vi "test-globallog for CSM error.vi"(8 "error in (no error)":errorcluster, 11 "TestCase in":refnum<class "testcase-globalLog.lvclass">) -> (0 "error out":errorcluster, 3 "TestCase out":refnum<class "testcase-globalLog.lvclass">)   [LabVIEW 2017, in "testcase-globalLog.lvclass"]
uses:
  testcase-globalLog.lvclass
  src/user.lib/_NEVSTOP/Communicable State Machine(CSM)/_Support/Priority Queue/Priority Queue.lvclass/Priority Queue.ctl
  src/user.lib/_NEVSTOP/Communicable State Machine(CSM)/_Support/Typedef/_CSM_GlobalLog_MSG.ctl
  src/user.lib/_NEVSTOP/Communicable State Machine(CSM)/_Support/Typedef/_CSM_Response Source Message.ctl
  src/user.lib/_NEVSTOP/Communicable State Machine(CSM)/_Support/Typedef/_CSM_GlobalLog_MSG_TYPE.ctl
  61f80922-628e-48dd-9b7e-09b6add618c8.vi
  src/user.lib/_NEVSTOP/Communicable State Machine(CSM)/_Support/GlobalEvent/Gevt-ThreadQueueName.vi
  src/user.lib/_NEVSTOP/Communicable State Machine(CSM)/_Support/Process/CSMP-Sync Call.vi
  src/user.lib/_NEVSTOP/Communicable State Machine(CSM)/Utility/uuid.vi
  src/user.lib/_NEVSTOP/Communicable State Machine(CSM)/Utility/Build Error Cluster.vi
  src/user.lib/_NEVSTOP/Communicable State Machine(CSM)/Utility/Trim Both Whitespace.vi
  src/user.lib/_NEVSTOP/Communicable State Machine(CSM)/_Support/CSMQ/_CSMObj-Message Check.vi
  src/user.lib/_NEVSTOP/Communicable State Machine(CSM)/_Support/CSMQ/_CSMObj-Enqueue Cross-Module Message.vi
  src/user.lib/_NEVSTOP/Communicable State Machine(CSM)/_Support/CSMQ/_CSMOFGV Get.vi
  src/user.lib/_NEVSTOP/Communicable State Machine(CSM)/_Support/Priority Queue/Enqueue Element.vi
  src/user.lib/_NEVSTOP/Communicable State Machine(CSM)/_Support/FGV-BroadcastRegistry/global-CSMQ FGV Change Flag.vi
  src/user.lib/_NEVSTOP/Communicable State Machine(CSM)/_Support/CSMQ/_CSMOFGV.vi
  src/user.lib/_NEVSTOP/Communicable State Machine(CSM)/_Support/Error/CSM No Target Error.vi
  src/user.lib/_NEVSTOP/Communicable State Machine(CSM)/_Support/Error/CSM Not Allowed Message.vi
  src/user.lib/_NEVSTOP/Communicable State Machine(CSM)/_Support/Error/CSM Target Error.vi
  src/user.lib/_NEVSTOP/Communicable State Machine(CSM)/_Support/Error/CSM Unhandled State Error.vi
  src/user.lib/_NEVSTOP/Communicable State Machine(CSM)/_Support/Error/CSM Target Timeout Error.vi
  <vilib>/addons/_JKI Toolkits/VI Tester/TestCase.llb/TestCase.lvclass
  src/user.lib/_NEVSTOP/Communicable State Machine(CSM)/Communicable State Machine.lvlib
  C:/Program Files (x86)/National Instruments/LabVIEW 2017/vi.lib/addons/_JKI Toolkits/VI Tester/TestCase.llb/TestCase.lvclass
panel:
  out "State History":string
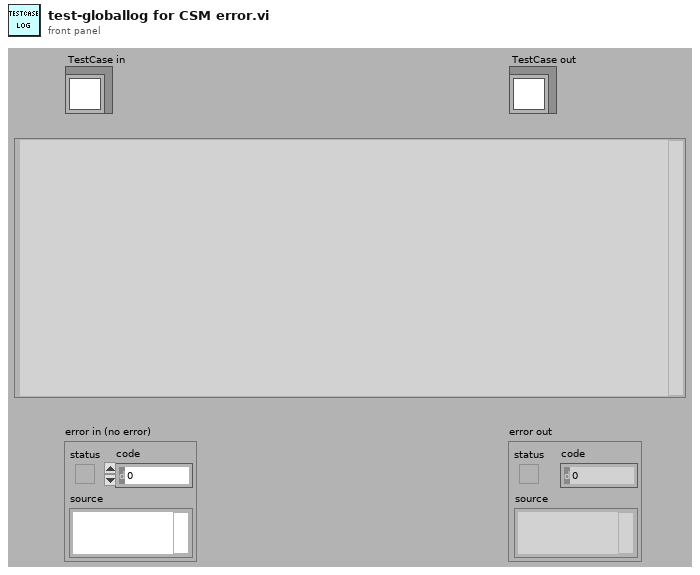
[diagram p1: front panel]
types:
  T1 = cluster{"threashold(#/s)":dbl, "Check Peroid(s)":dbl}
  T2 = typedef "Communicable State Machine.lvlib/_CSM_GlobalLog_MSG.ctl" = cluster{"Name(\"\" to use uuid)":string, "Current State":string, "Arguments":string, "Source Message":T3, "Source Module":string, "Complete(T)/Start(F)":bool, "LogType":T4}
  T3 = typedef "Communicable State Machine.lvlib/_CSM_Response Source Message.ctl" = cluster{"‘State":string, "’Arguments":string, "’Error":errorcluster}
  T4 = typedef "Communicable State Machine.lvlib/_CSM_GlobalLog_MSG_TYPE.ctl" = enum16{"User Log", "State Change", "Status", "Interrupt", "Register", "Unregister", "Error Log", "Module Created", "Module Destroyed"}
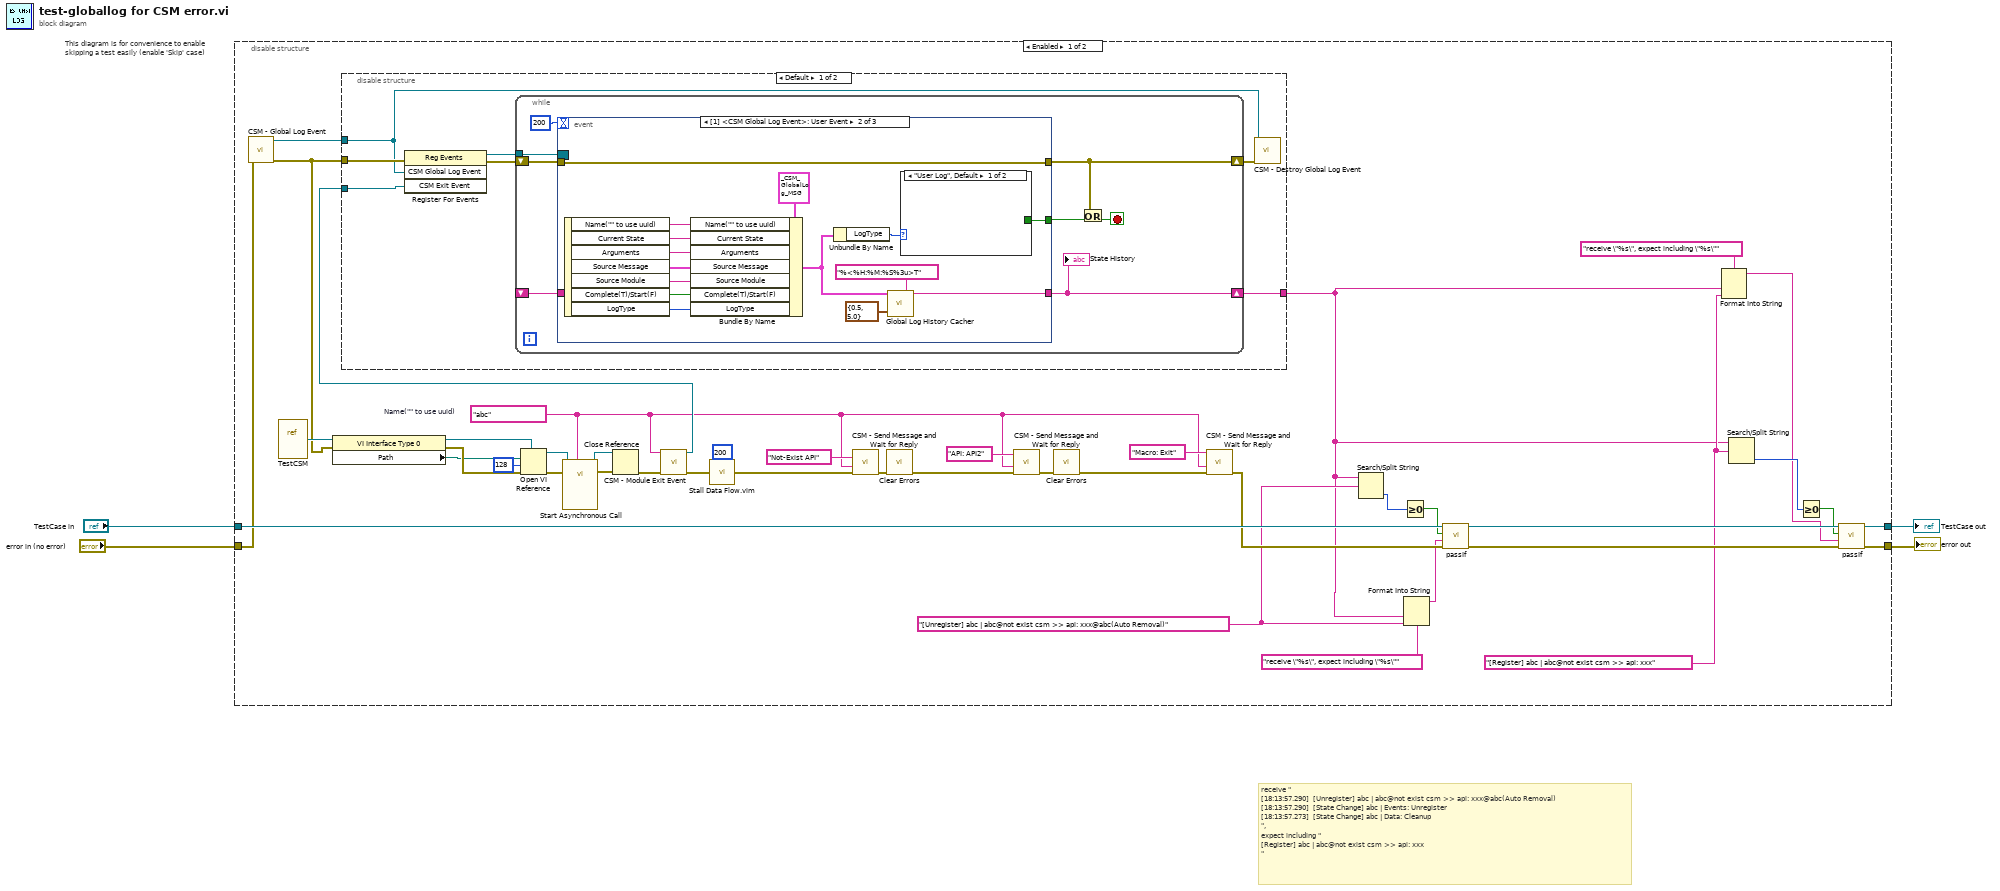
[diagram p0: block diagram]
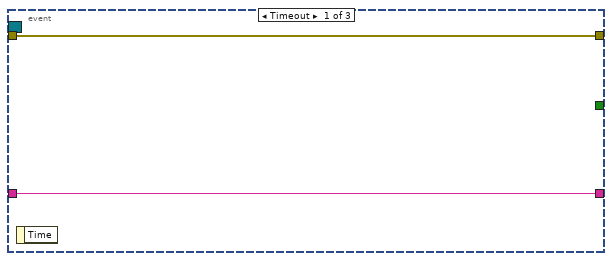
[diagram p2: hidden frame]
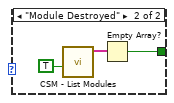
[diagram p3: hidden frame]
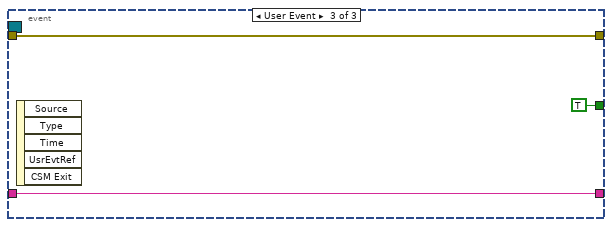
[diagram p4: hidden frame]
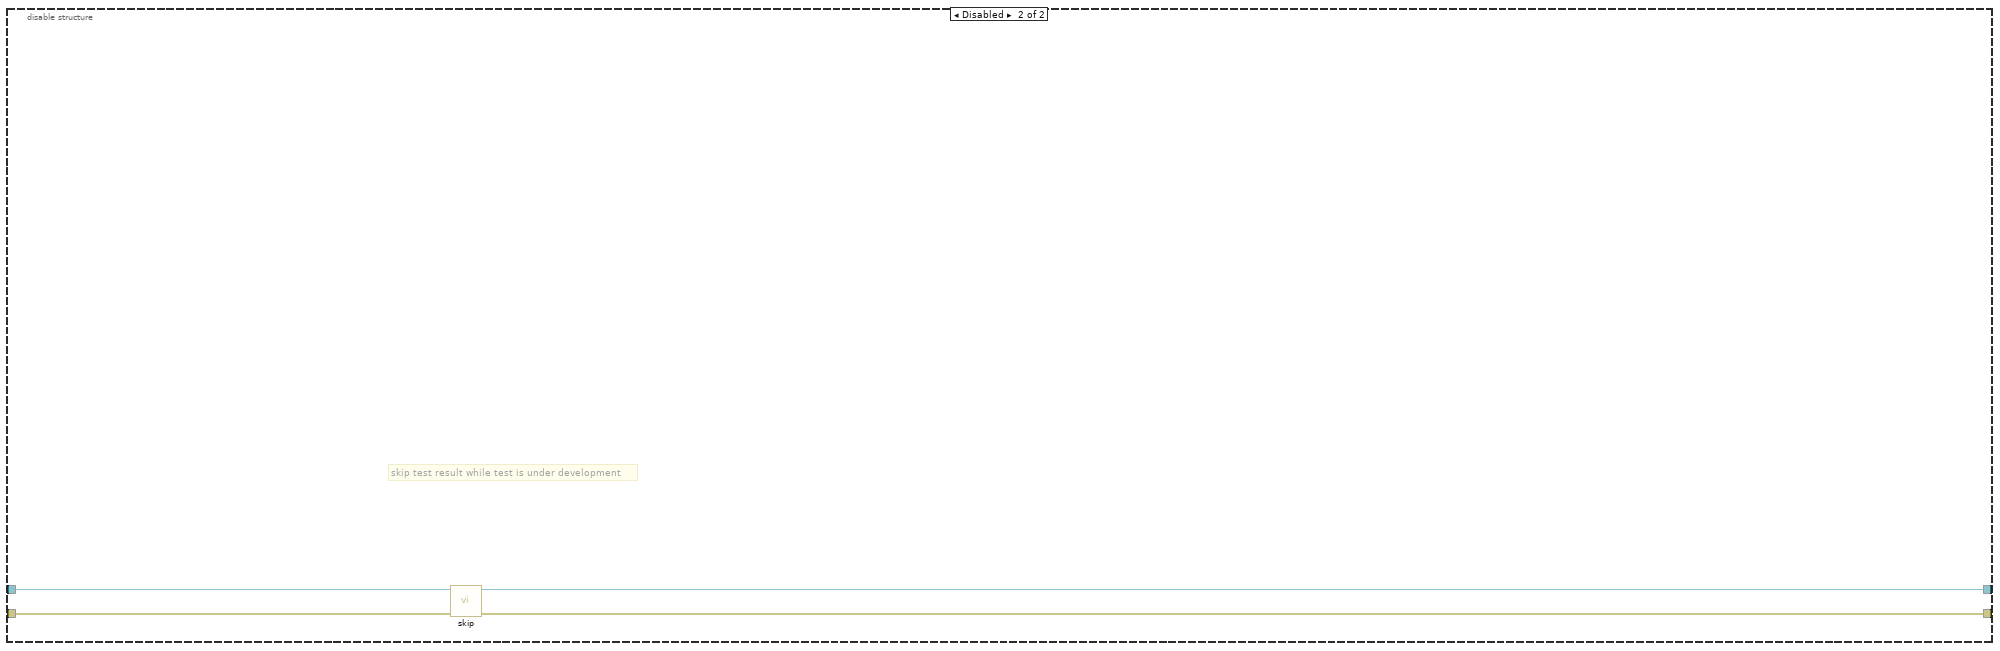
[diagram p6: hidden frame]
diagram:
  # "receive \"\n[18:13:57.290]  [Unregister] abc | abc@not exist csm >> api: xxx@abc(Auto Removal)\n[18:13:57.290]  [State Change] abc | Events: Unregister\n[18:13:57.273]  [State Change] abc | Data: Cleanup\n\", \nexpect including \"\n[Register] abc | abc@not exist csm >> api: xxx\n\""
  n1 = disable-structure "This diagram is for convenience to enable skipping a test easily (enable 'Skip' case)" shown="Enabled" {
    disable-tunnel: "TestCase in" -> [w46 w88]
    disable-tunnel: [w20 w86] -> w1
    disable-tunnel: [w19 w87] -> w3
    disable-tunnel: "error in (no error)" -> [w5 w85]
    frame Enabled {
      w10 = "[Register] abc | abc@not exist csm >> api: xxx" ("string")
      w13 = "[Unregister] abc | abc@not exist csm >> api: xxx@abc(Auto Removal)" ("string")
      w24 = "abc"  # Name("" to use uuid)
      n2 = call "CSM - Global Log Event.vi"("Error in"=w5) -> ("Error out"=w6:errorcluster, "CSM Global Log Event"=w7:refnum<user-event>)  [unwired: 9 in]
      n3 = vi-ref "TestCSM.vi"() -> (w38:refnum<vi>)
      n4 = property class="VI Interface Type 0"(reference=w38, error in=w6) -> (reference out=w42:refnum<vi>, error out=w40:errorcluster, "Path"=w39:path)
      n5 = Open VI Reference(type specifier VI Refnum (for type only)=w42, vi path=w39, options=128, error in (no error)=w40) -> (vi reference=w41:refnum<vi>, error out=w37:errorcluster)  [unwired: 2 in]
      n6 = call-by-ref "Start Asynchronous Call"(reference=w41, error in=w37, "Name(\"\" to use uuid)"=w24) -> (reference out=w44:refnum<vi>, error out=w43:errorcluster)  [unwired: 11 in]
      n7 = Close Reference(reference=w44, error in (no error)=w43) -> (error out=w36:errorcluster)
      n8 = call "CSM - Module Exit Event.vi"("Error in"=w36, "Name(\"\" to use uuid) in"=w24) -> ("Error out"=w35:errorcluster, "CSM Exit Event"=w34:refnum<user-event>)  [unwired: 8 in]
      n9 = disable-structure shown="Default" {
        disable-tunnel: w34 -> [w50 _]
        disable-tunnel: [w49 _] -> w8
        disable-tunnel: w6 -> [w48 _]
        disable-tunnel: w7 -> [w47 _]
        frame condition #0 (active) {
          n10 = register-events(error in=w48, w47, w50) -> (reference out=w52:refnum<event-registration>, error out=w53:errorcluster)  [unwired: 1 in]
          n11 = while {
            tunnel: w52 -> [w61]
            shift-right: [w58] -> w51
            shift-left: w53 -> [w60]
            shift-right: [w55] -> w49
            shift-left: _ -> [w54]
            stop <- w59 stop-if-true
            n12 = event shown="[1] <CSM Global Log Event>: User Event" {
              selector: w61 -> [_ _ _]
              dyn-events: _ -> [_ _ _]
              timeout: 200 -> [_ _ _]
              tunnel: w60 -> [w63 w78 w84]
              tunnel: [w63 w78 w84] -> w58
              tunnel: [_ w67 TRUE ("empty?")] -> w57
              tunnel: [w62 w64 w82] -> w55
              tunnel: w54 -> [w62 _ w82]
              event Timeout {
                n13 = event-data() -> ()  [unwired: 1 in, 1 out]
              }
              event User Event {
                n14 = event-data() -> ("Name(\"\" to use uuid)"=w77:string, "Current State"=w76:string, "Arguments"=w75:string, "Source Message"=w74:T3, "Source Module"=w73:string, "Complete(T)/Start(F)"=w72:bool, "LogType"=w71:T4)  [unwired: 1 in]
                n15 = Bundle By Name(cluster=T2 {"Name(\"\" to use uuid)"="", "Current State"="", "Arguments"="", "Source Message"={"‘State"="", "’Arguments"="", "’Error"={"status"=FALSE, "code"=0, "source"=""}}, "Source Module"="", "Complete(T)/Start(F)"=FALSE, "LogType"=enum."State Change"} ("Cross CSM Data"), "Name(\"\" to use uuid)"=w77, "Current State"=w76, "Arguments"=w75, "Source Message"=w74, "Source Module"=w73, "Complete(T)/Start(F)"=w72, "LogType"=w71) -> (w69:T2)
                n16 = Unbundle By Name(w69) -> ("LogType"=w68:T4)
                n17 = call "Global Log History Cacher.vi"("Cross CSM Data"=w69, "Time format string"="%<%H:%M:%S%3u>T", "Settings"=T1 {"threashold(#/s)"=0.5, "Check Peroid(s)"=5.0}) -> ("String Cache"=w64:string)  [unwired: 11 in, 1 out]
                n18 = case shown="\"User Log\", Default" w68 {
                  tunnel: [_ w79] -> w67
                  frame "User Log", Default {
                  }
                  frame "Module Destroyed" {
                    n19 = call "CSM - List Modules.vi"("All?"=TRUE) -> ("Module Names"=w81:string[])  [unwired: 9 in, 1 out]
                    n20 = Empty Array?(array=w81) -> (empty?=w79:bool)
                  }
                }
              }
              event User Event {
                n21 = event-data() -> ()  [unwired: 1 in, 5 out]
              }
            }
            "State History" <- w55
            n22 = Or(x=w58, y=w57) -> (x .or. y?=w59:bool)
          }
          n23 = call "CSM - Destroy Global Log Event.vi"("Error in"=w51, "CSM Global Log Event"=w47) -> ()  [unwired: 9 in, 1 out]
        }
        frame condition #1 {
        }
      }
      n24 = call "Stall Data Flow.vim"("value in"=w35, "milliseconds to wait"=u32 200) -> ("value out"=w30:errorcluster)  [unwired: 1 out]
      n25 = call "CSM - Send Message and Wait for Reply.vi"("Error In (no error)"=w30, "Target Module"=w24, "State"="Not-Exist API") -> ("error out"=w29:errorcluster)  [unwired: 6 in, 2 out]
      n26 = call <vilib>:"Clear Errors.vi"("error in (no error)"=w29) -> ("error out"=w25:errorcluster)  [unwired: 5 in, 1 out]
      n27 = call "CSM - Send Message and Wait for Reply.vi"("Error In (no error)"=w25, "Target Module"=w24, "State"="API: API2") -> ("error out"=w26:errorcluster)  [unwired: 6 in, 2 out]
      n28 = call <vilib>:"Clear Errors.vi"("error in (no error)"=w26) -> ("error out"=w23:errorcluster)  [unwired: 5 in, 1 out]
      n29 = call "CSM - Send Message and Wait for Reply.vi"("Error In (no error)"=w23, "Target Module"=w24, "State"="Macro: Exit") -> ("error out"=w33:errorcluster)  [unwired: 6 in, 2 out]
      n30 = Search/Split String(string=w8, search string/char (-)=w13) -> (offset of match=w18:i32)  [unwired: 1 in, 2 out]
      n31 = Greater Or Equal To 0?(x=w18) -> (x >= 0?=w17:bool)
      n32 = Format Into String(format string="receive \"%s\", expect including \"%s\"", w8, w13) -> (resulting string=w12:string)  [unwired: 2 in, 1 out]
      n33 = call-dynamic "passIf.vi"("error in (no error)"=w33, "message (\"\")"=w12, "pass"=w17, "TestCase in"=w46) -> ("error out"=w22:errorcluster, "TestCase out"=w21:refnum<class "testcase-globalLog.lvclass">)  [unwired: 6 in]
      n34 = Format Into String(format string="receive \"%s\", expect including \"%s\"", w8, w10) -> (resulting string=w9:string)  [unwired: 2 in, 1 out]
      n35 = Search/Split String(string=w8, search string/char (-)=w10) -> (offset of match=w16:i32)  [unwired: 1 in, 2 out]
      n36 = Greater Or Equal To 0?(x=w16) -> (x >= 0?=w15:bool)
      n37 = call-dynamic "passIf.vi"("error in (no error)"=w22, "message (\"\")"=w9, "pass"=w15, "TestCase in"=w21) -> ("error out"=w19:errorcluster, "TestCase out"=w20:refnum<class "testcase-globalLog.lvclass">)  [unwired: 6 in]
    }
    frame Disabled {
      # "skip test result while test is under development"
      n38 = call <vilib>:"skip.vi"("error in (no error)"=w85, "TestCase in"=w88) -> ("error out"=w87:errorcluster, "TestCase out"=w86:refnum<class "testcase-globalLog.lvclass">)  [unwired: 8 in]
    }
  }
  "error out" <- w3
  "TestCase out" <- w1
